vi "AutoCorrelation.vi"   [LabVIEW 2019, in "xy_utilities.lvlib"]
doc: "Compute the autocorrelation <b>R_aa</b> of <b>XY-data a</b>.\n\nWire data to the data input to determine the polymorphic instance to use or manually select the instance."
uses:
  xy_utilities.lvlib
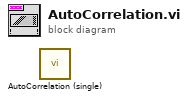
[diagram p0: block diagram]
diagram:
  n1 = call "AutoCorrelation (single).vi"() -> ()  [unwired: 10 in, 2 out]
